vi "CRYUnflatten CDD Sub.vi"(10 "Flatten Data In":string) -> (0 "error out":errorcluster, 3 "Converted CDD":string)   [LabVIEW 2013]
panel:
  out "CDD Out":T1 {"Data Cluster"."Results"."Margin" format="%.2f"; "Data Cluster"."Waveforms"."Y dB ref" format="%.1f"; "Data Cluster"."Waveforms"."Y axis" items=["Log", "Lin"]; "Data Cluster"."Waveforms"."Y data" items=["dB", "Lin"]; "Data Cluster"."Waveforms"."X data" items=["dB", "Lin"]; "Data Cluster"."Values"."Z data" items=["dB", "Lin"]; "Data Cluster"."Values"."X data" items=["dB", "Lin"]; "Data Cluster"."Values"."Y data" items=["dB", "Lin"]; "Data Cluster"."Values"."Z dB ref" format="%.1f"; "Data Cluster"."Values"."Z axis" items=["Log", "Lin"]; "Data Cluster"."Values"."X dB ref" format="%.1f"; "Data Cluster"."Values"."X axis" items=["Log", "Lin"]; "Data Cluster"."Values"."Y axis" items=["Log", "Lin"]; "Data Cluster"."Values"."Y dB ref" format="%.1f"; "Data Cluster"."Values"."Curve"."z" format="%.2f"; "Data Cluster"."Values"."Curve"."y" format="%.2f"; "Data Cluster"."Values"."Curve"."x" format="%.2f"; "Data Cluster"."Curves"."Z data" items=["dB", "Lin"]; "Data Cluster"."Curves"."X data" items=["dB", "Lin"]; "Data Cluster"."Curves"."Y data" items=["dB", "Lin"]; "Data Cluster"."Curves"."Z dB ref" format="%.1f"; "Data Cluster"."Curves"."Z axis" items=["Log", "Lin"]; "Data Cluster"."Curves"."X dB ref" format="%.1f"; "Data Cluster"."Curves"."X axis" items=["Log", "Lin"]; "Data Cluster"."Curves"."Y axis" items=["Log", "Lin"]; "Data Cluster"."Curves"."Y dB ref" format="%.1f"; "Data Cluster"."Curves"."Curve"."z" format="%.2f"; "Data Cluster"."Curves"."Curve"."y" format="%.2f"; "Data Cluster"."Curves"."Curve"."x" format="%.2f"}
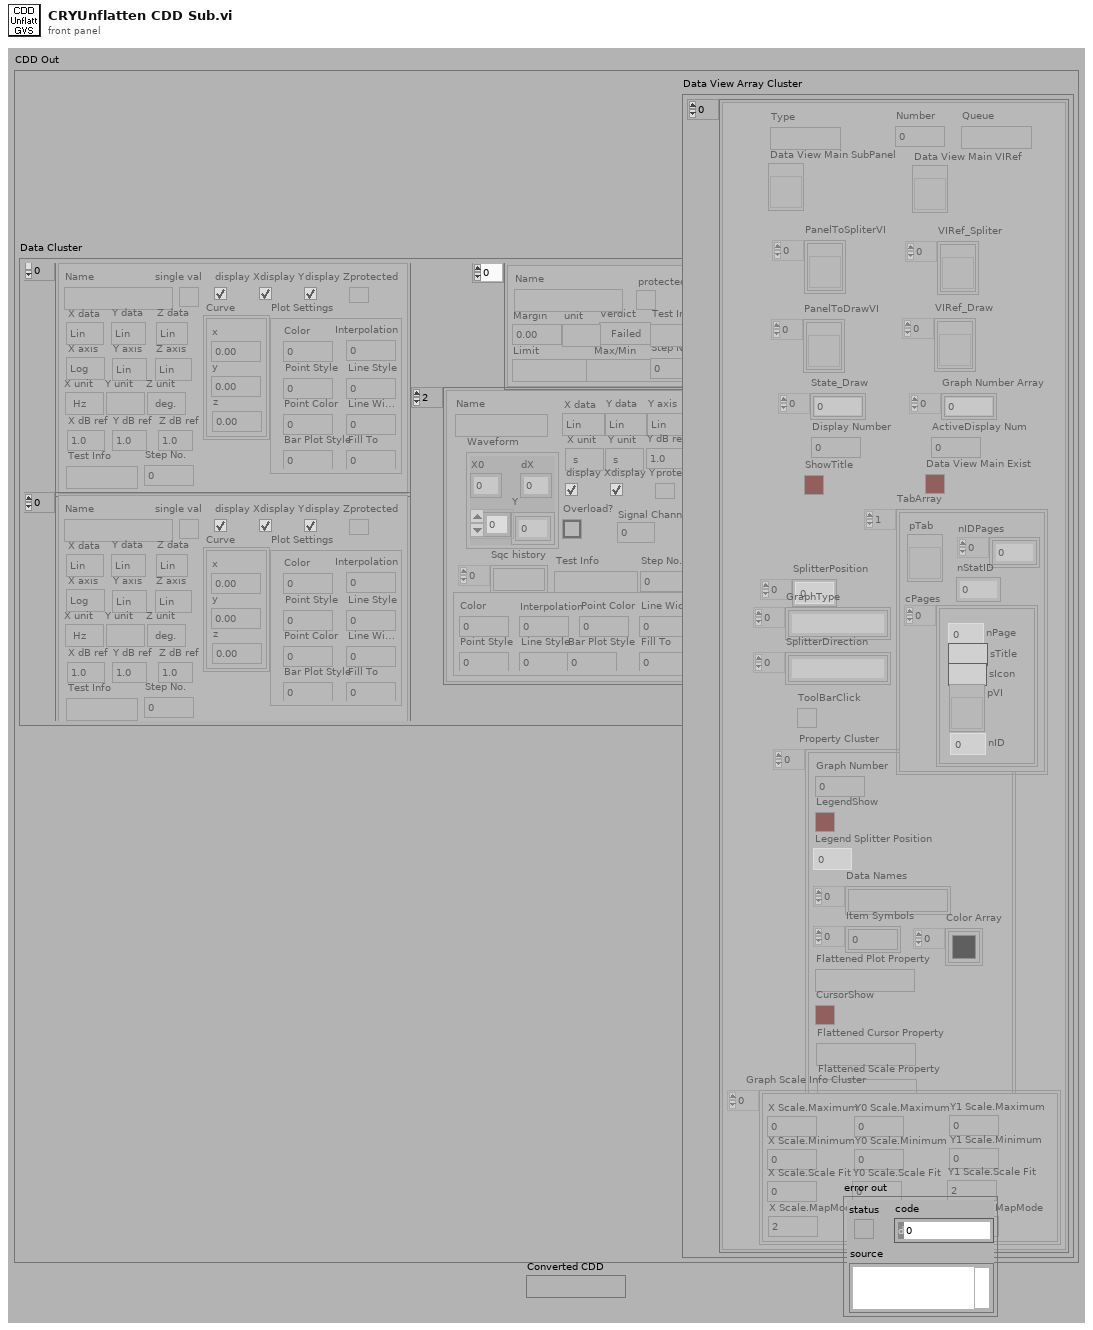
[diagram p1: front panel]
types:
  T1 = cluster{"Data Cluster":cluster{"Curves":cluster{"Name":string, "Curve":cluster{"x":dbl, "y":dbl, "z":dbl}[], "X data":u16, "Y data":u16, "Z data":u16, "X axis":u16, "Y axis":u16, "Z axis":u16, "X unit":string, "Y unit":string, "Z unit":string, "X dB ref":dbl, "Y dB ref":dbl, "Z dB ref":dbl, "single val":bool, "protected":bool, "display X":bool, "display Y":bool, "display Z":bool, "Test Info":string, "Step No.":u16, "Plot Settings":cluster{"Color":u32, "Interpolation":u8, "Point Style":u8, "Line Style":u8, "Point Color":u32, "Line Width":u8, "Bar Plot Style":u8, "Fill To":i16}}[], "Values":cluster{"Name":string, "Curve":cluster{"x":dbl, "y":dbl, "z":dbl}[], "X data":u16, "Y data":u16, "Z data":u16, "X axis":u16, "Y axis":u16, "Z axis":u16, "X unit":string, "Y unit":string, "Z unit":string, "X dB ref":dbl, "Y dB ref":dbl, "Z dB ref":dbl, "single val":bool, "protected":bool, "display X":bool, "display Y":bool, "display Z":bool, "Test Info":string, "Step No.":u16, "Plot Settings":cluster{"Color":u32, "Interpolation":u8, "Point Style":u8, "Line Style":u8, "Point Color":u32, "Line Width":u8, "Bar Plot Style":u8, "Fill To":i16}}[], "Results":cluster{"Name":string, "Margin":dbl, "unit":string, "Verdict":bool, "Limit":string, "Max/Min":string, "protected":bool, "Step No.":u16, "Test Info":string}[], "Waveforms":cluster{"Waveform":cluster{"X0":dbl, "dX":dbl, "Y":sgl[]}, "X data":u16, "Y data":u16, "Y axis":u16, "X unit":string, "Y unit":string, "Y dB ref":dbl, "display Y":bool, "display X":bool, "Overload?":bool, "Test Info":string, "Step No.":u16, "Name":string, "protected":bool, "Sqc history":string[], "Signal Channel ID":i32, "Plot Settings":cluster{"Color":u32, "Interpolation":u8, "Point Style":u8, "Line Style":u8, "Point Color":u32, "Line Width":u8, "Bar Plot Style":u8, "Fill To":i16}}[]}, "Data View Array Cluster":cluster{"Data View Array":cluster{"Data View Main Exist":bool, "Data View Main SubPanel":refnum<vi>, "PanelToSpliterVI":refnum<vi>[], "VIRef_Spliter":refnum<vi>[], "VIRef_Draw":refnum<vi>[], "PanelToDrawVI":refnum<vi>[], "State_Draw":i8[], "Graph Number Array":i32[], "Display Number":i32, "ActiveDisplay Num":i32, "ShowTitle":bool, "Data View Main VIRef":refnum<vi>, "Type":string, "Number":i32, "Queue":string, "Property Cluster":cluster{"LegendShow":bool, "Legend Splitter Position":dbl, "Data Names":string[], "Item Symbols":i32[], "Color Array":u32[], "Flattened Plot Property":string, "CursorShow":bool, "Flattened Cursor Property":string, "Graph Number":i32, "Flattened Scale Property":string}[], "SplitterPosition":dbl[], "GraphType":string[], "SplitterDirection":string[], "Graph Scale Info Cluster":cluster{"X Scale.Maximum":dbl, "X Scale.Minimum":dbl, "X Scale.Scale Fit":u8, "Y0 Scale.Maximum":dbl, "Y0 Scale.Minimum":dbl, "Y0 Scale.Scale Fit":u8, "Y1 Scale.Maximum":dbl, "Y1 Scale.Minimum":dbl, "Y1 Scale.Scale Fit":u8, "X Scale.MapMode":u8, "Y1 Scale.MapMode":u8, "Y0 Scale.MapMode":u8}[], "TabArray":cluster{"cPages":cluster{"nPage":i32, "sTitle":string, "sIcon":string, "pVI":refnum<vi>, "nID":i32}[], "pTab":refnum<vi>, "nIDPages":i32[], "nStatID":i32}[], "ToolBarClick":bool}[]}}
  T2 = cluster{"Data Cluster":cluster{"Curves":cluster{"Name":string, "Curve":cluster{"x":dbl, "y":dbl, "z":dbl}[], "X data":u16, "Y data":u16, "Z data":u16, "X axis":u16, "Y axis":u16, "Z axis":u16, "X unit":string, "Y unit":string, "Z unit":string, "X dB ref":dbl, "Y dB ref":dbl, "Z dB ref":dbl, "single val":bool, "protected":bool, "display X":bool, "display Y":bool, "display Z":bool, "Test Info":string, "Step No.":u16, "Plot Settings":cluster{"Color":u32, "Interpolation":u8, "Point Style":u8, "Line Style":u8, "Point Color":u32, "Line Width":u8, "Bar Plot Style":u8, "Fill To":i16}}[], "Values":cluster{"Name":string, "Curve":cluster{"x":dbl, "y":dbl, "z":dbl}[], "X data":u16, "Y data":u16, "Z data":u16, "X axis":u16, "Y axis":u16, "Z axis":u16, "X unit":string, "Y unit":string, "Z unit":string, "X dB ref":dbl, "Y dB ref":dbl, "Z dB ref":dbl, "single val":bool, "protected":bool, "display X":bool, "display Y":bool, "display Z":bool, "Test Info":string, "Step No.":u16, "Plot Settings":cluster{"Color":u32, "Interpolation":u8, "Point Style":u8, "Line Style":u8, "Point Color":u32, "Line Width":u8, "Bar Plot Style":u8, "Fill To":i16}}[], "Results":cluster{"Name":string, "Margin":dbl, "unit":string, "Verdict":bool, "Limit":string, "Max/Min":string, "protected":bool, "Step No.":u16, "Test Info":string}[], "Waveforms":cluster{"Waveform":cluster{"X0":dbl, "dX":dbl, "Y":sgl[]}, "X data":u16, "Y data":u16, "Y axis":u16, "X unit":string, "Y unit":string, "Y dB ref":dbl, "display Y":bool, "display X":bool, "Overload?":bool, "Test Info":string, "Step No.":u16, "Name":string, "protected":bool, "Sqc history":string[], "Signal Channel ID":i32, "Plot Settings":cluster{"Color":u32, "Interpolation":u8, "Point Style":u8, "Line Style":u8, "Point Color":u32, "Line Width":u8, "Bar Plot Style":u8, "Fill To":i16}}[]}, "Data View Array Cluster":cluster{"Data View Array":cluster{"Data View Main Exist":bool, "Data View Main SubPanel":refnum<vi>, "PanelToSpliterVI":refnum<vi>[], "VIRef_Spliter":refnum<vi>[], "VIRef_Draw":refnum<vi>[], "PanelToDrawVI":refnum<vi>[], "State_Draw":i8[], "Graph Number Array":i32[], "Display Number":i32, "ActiveDisplay Num":i32, "ShowTitle":bool, "Data View Main VIRef":refnum<vi>, "Type":string, "Number":i32, "Queue":string, "Property Cluster":cluster{"LegendShow":bool, "Legend Splitter Position":dbl, "Data Names":string[], "Item Symbols":i32[], "Color Array":u32[], "Flattened Plot Property":string, "CursorShow":bool, "Flattened Cursor Property":string}[], "SplitterPosition":dbl[], "GraphType":string[], "SplitterDirection":string[], "Graph Scale Info Cluster":cluster{"X Scale.Maximum":dbl, "X Scale.Minimum":dbl, "X Scale.Scale Fit":u8, "Y0 Scale.Maximum":dbl, "Y0 Scale.Minimum":dbl, "Y0 Scale.Scale Fit":u8, "Y1 Scale.Maximum":dbl, "Y1 Scale.Minimum":dbl, "Y1 Scale.Scale Fit":u8, "X Scale.MapMode":u8, "Y1 Scale.MapMode":u8, "Y0 Scale.MapMode":u8}[], "TabArray":cluster{"cPages":cluster{"nPage":i32, "sTitle":string, "sIcon":string, "pVI":refnum<vi>, "nID":i32}[], "pTab":refnum<vi>, "nIDPages":i32[], "nStatID":i32}[], "ToolBarClick":bool}[]}}
  T3 = cluster{"unsigned byte array[0]":u8, "unsigned byte array[1]":u8, "unsigned byte array[2]":u8}
  T4 = typedef "CRYCurve Library Cluster.ctl" = cluster{"Curves":T5, "Results":T7, "Values":T5, "Waveforms":T9, "Curve Items":cluster{"Left Cell String":string, "Child Text":string[], "Child Tag":string, "Item Indent":i32, "Child Only?":bool, "Glyph Index":i32}[], "Value Items":cluster{"Left Cell String":string, "Child Text":string[], "Child Tag":string, "Item Indent":i32, "Child Only?":bool, "Glyph Index":i32}[], "Result Items":cluster{"Left Cell String":string, "Child Text":string[], "Child Tag":string, "Item Indent":i32, "Child Only?":bool, "Glyph Index":i32}[], "WFM Items":cluster{"Left Cell String":string, "Child Text":string[], "Child Tag":string, "Item Indent":i32, "Child Only?":bool, "Glyph Index":i32}[]}
  T5 = typedef "CRYData Cluster Array.ctl" = T6[]
  T6 = typedef "CRYData Cluster.ctl" = cluster{"Name":string, "Curve":cluster{"x":dbl, "y":dbl, "z":dbl}[], "X data":u16, "Y data":u16, "Z data":u16, "X axis":u16, "Y axis":u16, "Z axis":u16, "X unit":string, "Y unit":string, "Z unit":string, "X dB ref":dbl, "Y dB ref":dbl, "Z dB ref":dbl, "single val":bool, "protected":bool, "display X":bool, "display Y":bool, "display Z":bool, "Test Info":string, "Step No.":i32, "Plot Settings":cluster{"Color":u32, "Interpolation":u8, "Point Style":u8, "Line Style":u8, "Point Color":u32, "Line Width":u8, "Bar Plot Style":u8, "Fill To":i16}, "AutoProtect":bool}
  T7 = typedef "CRYResult Cluster Array.ctl" = T8[]
  T8 = typedef "CRYResult Cluster.ctl" = cluster{"Name":string, "Margin":dbl, "unit":string, "Verdict":bool, "Limit":string, "Max/Min":string, "protected":bool, "Step No.":i32, "Test Info":string, "AutoProtect":bool}
  T9 = typedef "CRYWaveform Cluster Array.ctl" = T10[]
  T10 = typedef "CRYWaveform Cluster.ctl" = cluster{"Waveform":cluster{"X0":dbl, "dX":dbl, "Y":sgl[]}, "X data":u16, "Y data":u16, "Y axis":u16, "X unit":string, "Y unit":string, "Y dB ref":dbl, "display Y":bool, "display X":bool, "Overload?":bool, "Test Info":string, "Step No.":i32, "Name":string, "protected":bool, "Sqc history":string[], "Signal Channel ID":i32, "Plot Settings":cluster{"Color":u32, "Interpolation":u8, "Point Style":u8, "Line Style":u8, "Point Color":u32, "Line Width":u8, "Bar Plot Style":u8, "Fill To":i16}, "AutoProtect":bool}
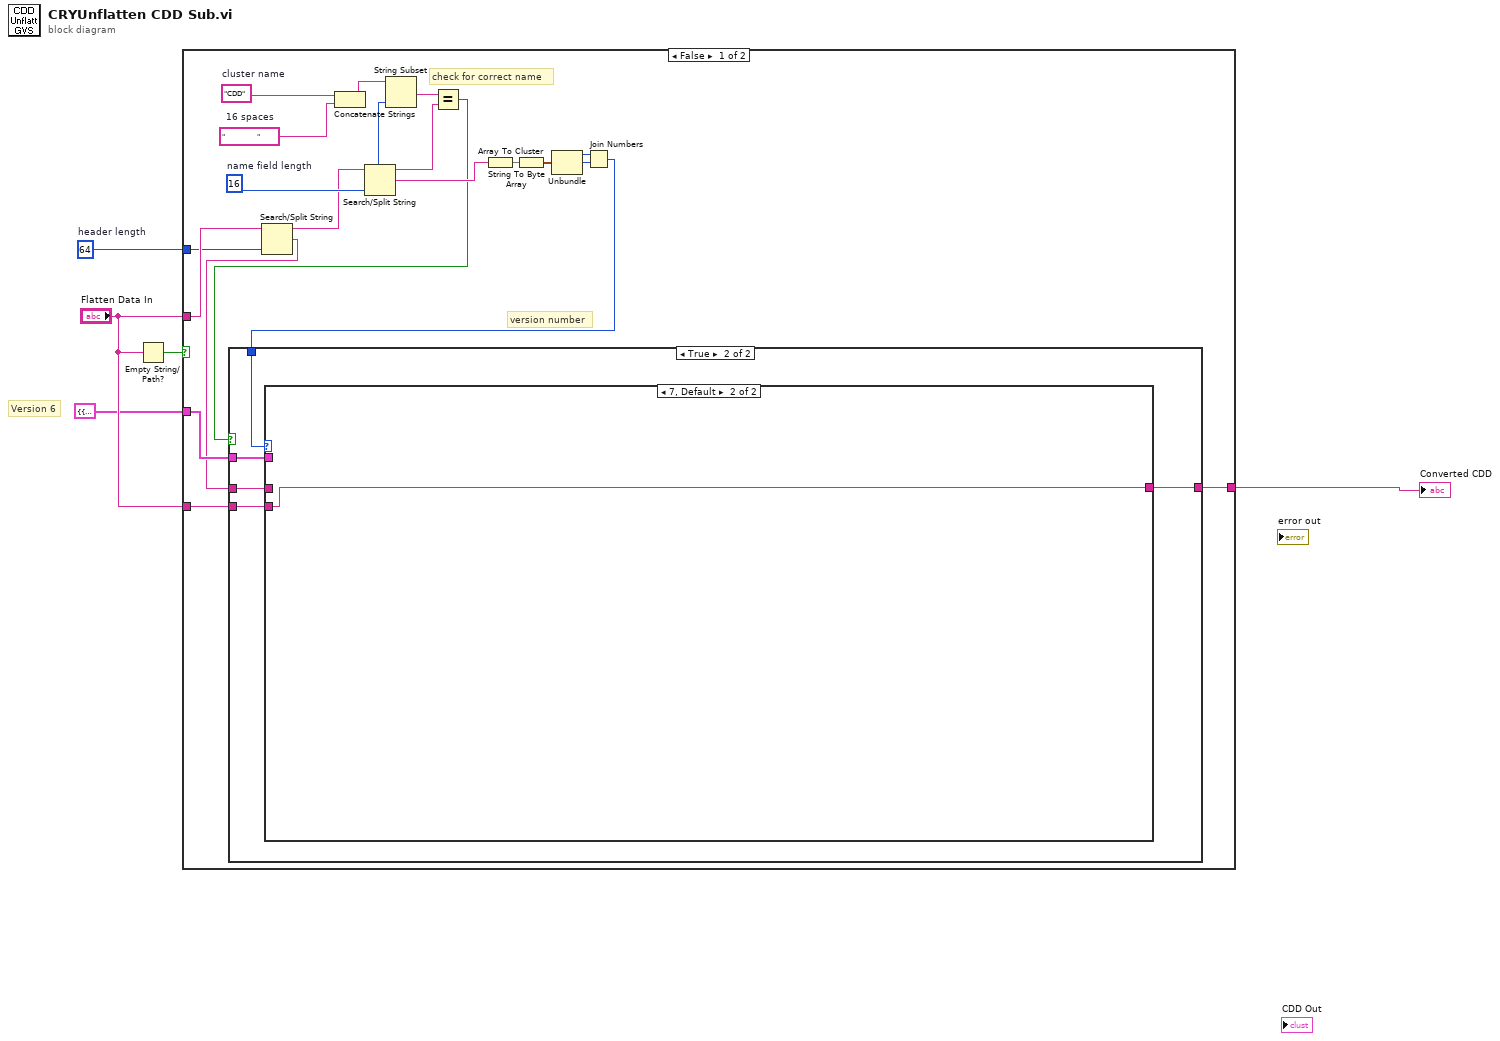
[diagram p0: block diagram]
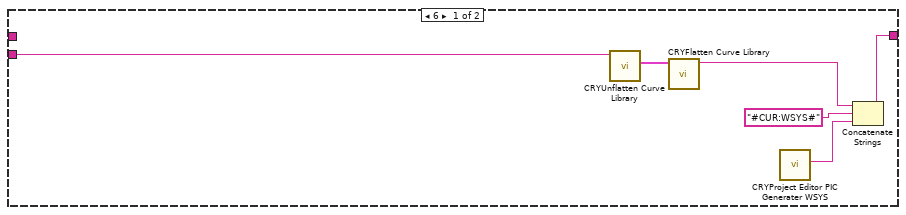
[diagram p3: hidden frame]
diagram:
  w4 = 64  # header length
  # "Version 6"
  n1 = Empty String/Path?(string/path="Flatten Data In") -> (empty?=w5:bool)
  n2 = case shown="False" w5 {
    tunnel: "Flatten Data In" -> [w12 w39]
    tunnel: T2 {"Data Cluster"={"Curves"=[], "Values"=[], "Results"=[], "Waveforms"=[]}, "Data View Array Cluster"={"Data View Array"=[]}} ("CDD Out") -> [w25 _]
    tunnel: w4 -> [w11 _]
    tunnel: "Flatten Data In" -> [w8 _]
    tunnel: [w6 w39] -> w1
    frame False {
      w20 = "                "  # 16 spaces
      w19 = "CDD"  # cluster name
      w22 = 16  # name field length
      # "check for correct name"
      # "version number"
      n3 = Search/Split String(string=w12, offset (0)=w11) -> (substring before match=w17:string, match + rest of string=w7:string)  [unwired: 2 out]
      n4 = Concatenate Strings(w19, w20) -> (w21:string)
      n5 = Search/Split String(string=w17, offset (0)=w22) -> (substring before match=w24:string, match + rest of string=w18:string)  [unwired: 2 out]
      n6 = String Subset(string=w21, length (rest)=w22) -> (substring=w23:string)  [unwired: 1 out]
      n7 = Equal?(x=w23, y=w24) -> (x = y?=w10:bool)
      n8 = String To Byte Array(string=w18) -> (unsigned byte array=w13:u8[])
      n9 = Array To Cluster(array=w13) -> (cluster=w14:T3)
      n10 = Unbundle(w14) -> ("unsigned byte array[0]"=w15:u8, "unsigned byte array[1]"=w16:u8)  [unwired: 1 out]
      n11 = Join Numbers(hi=w15, lo=w16) -> ((hi.lo)=w9:u16)
      n12 = case shown="True" w10 {
        tunnel: w25 -> [_ w31]
        tunnel: w9 -> [_ w30]
        tunnel: w8 -> [w26 w29]
        tunnel: w7 -> [_ w28]
        tunnel: [w26 w27] -> w6
        frame False {
        }
        frame True {
          n13 = case shown="7, Default" w30 {
            tunnel: w31 -> [_ _]
            tunnel: w29 -> [w33 w38]
            tunnel: [w35 w38] -> w27
            tunnel: w28 -> [_ _]
            frame 6 {
              n14 = call "CRYUnflatten Curve Library.vi"("Flatten CurLib"=w33) -> ("CurLib Cluster"=w32:T4)  [unwired: 8 in, 2 out]
              n15 = call "CRYFlatten Curve Library.vi"("CurLibData"=w32) -> ("CurLib flattened"=w36:string)  [unwired: 10 in]
              n16 = call "CRYProject Editor PIC Generater WSYS.vi"() -> ("sData_Out"=w34:string)  [unwired: 11 in]
              n17 = Concatenate Strings(w36, "#CUR:WSYS#", w34) -> (w35:string)
            }
            frame 7, Default {
            }
          }
        }
      }
    }
    frame True {
    }
  }
  "Converted CDD" <- w1
